vi "lfieldpanel_DO_acquire_single_frame.vi"(5 "savepath":path, 7 "Log data":bool, 8 "error in (no error)":errorcluster, 9 "notes":string, 10 "Integrate_sensor":bool, 11 "lightfield_panel in":refnum<class "lightfield_panel.lvclass">) -> (0 "error out":errorcluster, 3 "lightfield_panel out":refnum<class "lightfield_panel.lvclass">)   [LabVIEW 2015, in "lightfield_panel.lvclass"]
uses:
  lightfield_panel.lvclass
  lightfield/lightfield_class.lvclass
  UI/panel_class/panel.lvclass
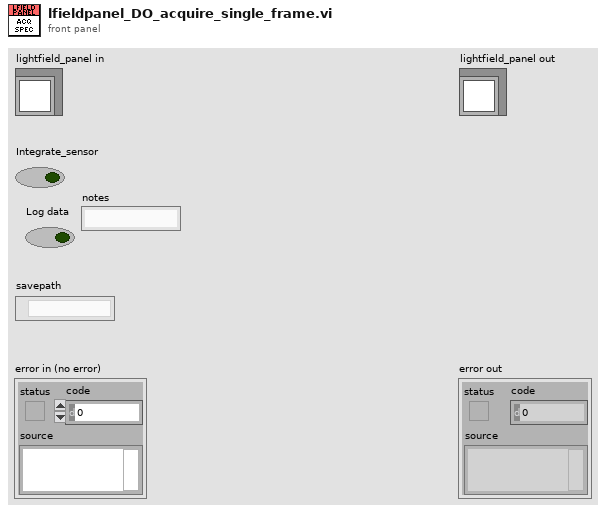
[diagram p1: front panel]
types:
  T1 = cluster{"Image":dbl[][][], "Frame Size":cluster{"F":i32, "Y":i32, "X":i32}}
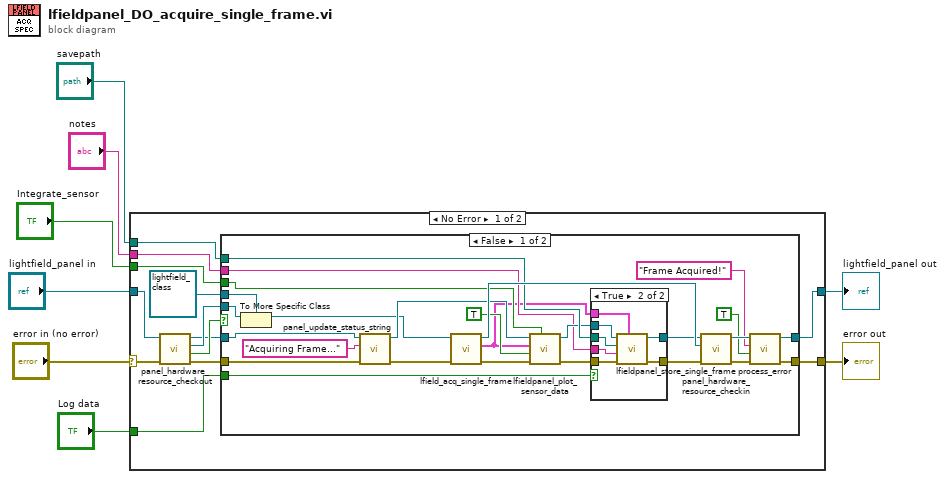
[diagram p0: block diagram]
diagram:
  n1 = case shown="No Error" "error in (no error)" {
    selector: "error in (no error)" -> [w21 w60]
    tunnel: [w15 w60] -> w5
    tunnel: [w14 w59] -> w7
    tunnel: "lightfield_panel in" -> [w13 w59]
    tunnel: "Integrate_sensor" -> [w12 _]
    tunnel: "Log data" -> [w11 _]
    tunnel: "savepath" -> [w10 _]
    tunnel: "notes" -> [w9 _]
    frame No Error {
      n2 = call "panel_hardware_resource_checkout.vi"("error in (no error)"=w21, "panel in"=w13) -> ("error out"=w17:errorcluster, "timed out?"=w20:bool, "hardware.lvclass"=w18:refnum<class "hardware.lvclass">, "panel out"=w16:refnum<class "lightfield_panel.lvclass">)  [unwired: 6 in]
      n3 = case shown="False" w20 {
        tunnel: refnum<class "lightfield_class.lvclass"> refnum ("lightfield_class.lvclass") -> [w47 _]
        tunnel: w18 -> [w46 _]
        tunnel: w17 -> [w35 w57]
        tunnel: w16 -> [w33 w58]
        tunnel: [w43 w57] -> w15
        tunnel: [w42 w58] -> w14
        tunnel: w12 -> [w37 _]
        tunnel: w11 -> [w31 _]
        tunnel: w10 -> [w29 _]
        tunnel: w9 -> [w25 _]
        frame False {
          n4 = To More Specific Class(target class=w47, reference=w46) -> (specific class reference=w23:refnum<class "lightfield_class.lvclass">)  [unwired: 1 in, 1 out]
          n5 = call-dynamic "panel_update_status_string.vi"("error in (no error)"=w35, "String"="Acquiring Frame...", "lightfield_panel in"=w33) -> ("error out"=w22:errorcluster, "lightfield_panel out"=w34:refnum<class "lightfield_panel.lvclass">)  [unwired: 7 in]
          n6 = call "lfield_acq_single_frame.vi"("error in (no error)"=w22, "lightfield_class in"=w23) -> ("error out"=w38:errorcluster, "image_data"=w24:T1, "lightfield_class out"=w39:refnum<class "lightfield_class.lvclass">)  [unwired: 7 in]
          n7 = call "lfieldpanel_plot_sensor_data.vi"("Integrate"=w37, "error in (no error)"=w38, "First_time?"=TRUE, "image_data"=w24, "lightfield_panel in"=w34) -> ("error out"=w30:errorcluster, "lightfield_panel out"=w27:refnum<class "lightfield_panel.lvclass">)  [unwired: 5 in]
          n8 = case shown="True" w31 {
            tunnel: w30 -> [w49 w56]
            tunnel: w29 -> [_ w52]
            tunnel: [w49 w55] -> w28
            tunnel: w27 -> [w48 w54]
            tunnel: [w48 w53] -> w26
            tunnel: w25 -> [_ w51]
            tunnel: w24 -> [_ w50]
            frame False {
            }
            frame True {
              n9 = call "lfieldpanel_store_single_frame.vi"("image_data"=w50, "error in (no error)"=w56, "notes"=w51, "Path"=w52, "lightfield_panel in"=w54) -> ("error out"=w55:errorcluster, "lightfield_panel out"=w53:refnum<class "lightfield_panel.lvclass">)  [unwired: 5 in]
            }
          }
          n10 = call "panel_hardware_resource_checkin.vi"("error in (no error)"=w28, "hardware.lvclass"=w39, "panel in"=w26) -> ("error out"=w44:errorcluster, "panel out"=w45:refnum<class "lightfield_panel.lvclass">)  [unwired: 7 in]
          n11 = call "process_error.vi"("error in (no error)"=w44, "Update Status"=TRUE, "No Error Message"="Frame Acquired!", "lightfield_panel in"=w45) -> ("error out"=w43:errorcluster, "lightfield_panel out"=w42:refnum<class "lightfield_panel.lvclass">)  [unwired: 6 in]
        }
        frame True {
        }
      }
    }
    frame Error {
    }
  }
  "error out" <- w5
  "lightfield_panel out" <- w7
